vi "Abort Recipe.vi"(8 "error in (no error)":errorcluster, 11 "Recipe Process in":refnum<class "Recipe Process.lvclass">) -> (0 "error out":errorcluster, 3 "Recipe Process out":refnum<class "Recipe Process.lvclass">)   [LabVIEW 2022 SP3, in "Recipe Process.lvlib" / "Recipe Process.lvclass"]
uses:
  Recipe Process.lvclass
  Recipe Process.lvclass/Recipe Process.ctl
  XY Stage/Process Actor/Process Framework/Process State Data/Process State Data.lvclass
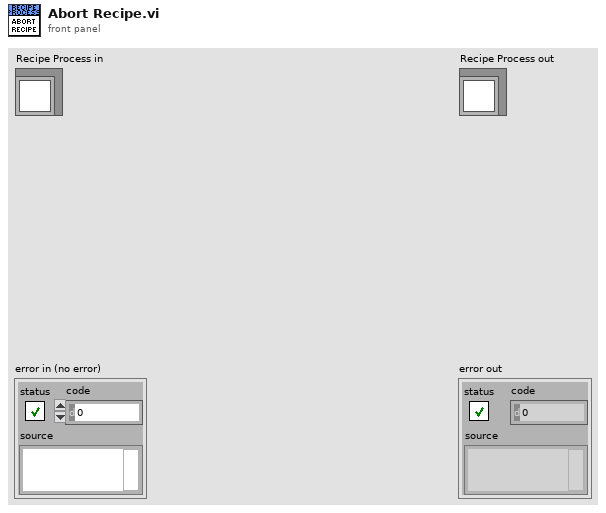
[diagram p1: front panel]
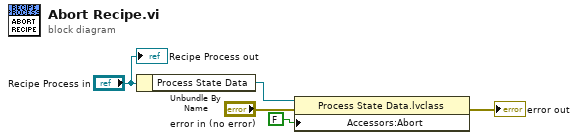
[diagram p0: block diagram]
diagram:
  n1 = Unbundle By Name("Recipe Process in") -> ("Process State Data"=w4:refnum<data-value>)
  n2 = property class="Process State Data.lvclass"(reference=w4, error in="error in (no error)", "Accessors:Abort"=FALSE ("Abort")) -> (error out=→"error out":errorcluster)  [unwired: 1 out]
  "Recipe Process out" <- "Recipe Process in"
